vi "GraphView.vi"(1 "Increment":dbl, 2 "End":dbl, 3 "Start":dbl) -> (0 "Array":dbl[](array[numeric]))   [LabVIEW 2023]
panel:
  out "increment":dbl format="%#_4f"
  in  "stop":bool
  out "Waveform Graph":dbl[][](graph)
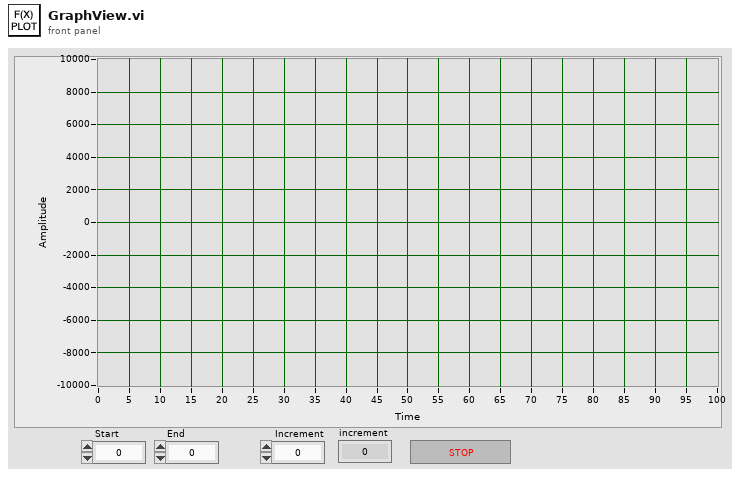
[diagram p1: front panel]
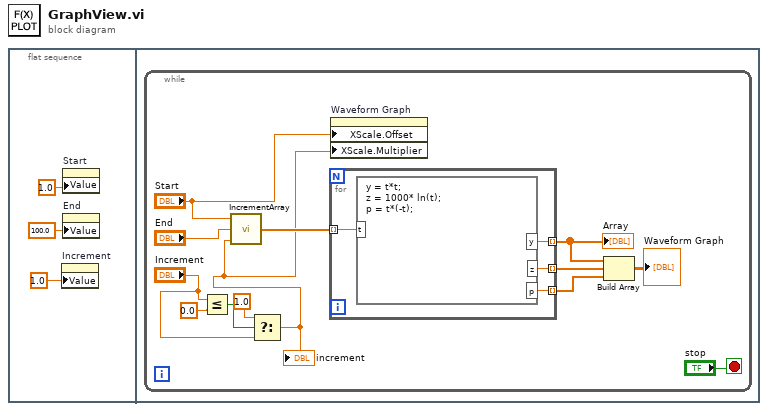
[diagram p0: block diagram]
diagram:
  n1 = flat-sequence {
    frame #0 {
      n2 = property on="Increment" class="DigNum (strict)"("Value"=1.0 ("End")) -> ()  [unwired: 2 in, 2 out]
      n3 = property on="Start" class="DigNum (strict)"("Value"=1.0 ("Start")) -> ()  [unwired: 2 in, 2 out]
      n4 = property on="End" class="DigNum (strict)"("Value"=100.0 ("End")) -> ()  [unwired: 2 in, 2 out]
    }
    frame #1 {
      n5 = while {
        stop <- "stop" stop-if-true
        n6 = Less Or Equal?(x="Increment", y=0.0) -> (x <= y?=w7:bool)
        n7 = Select(t=1.0, s=w7, f="Increment") -> (s? t:f=w4:dbl)
        "increment" <- w4
        n8 = call "IncrementArray.vi"("Increment"=w4, "End"="End", "Start"="Start") -> ("Array"=w15:dbl[])
        n9 = for {
          tunnel: w15 -> [w19] mode=indexing
          tunnel: [w20] -> w13 mode=indexing
          tunnel: [w18] -> w12 mode=indexing
          tunnel: [w17] -> w10 mode=indexing
          n10 = formula code="y = t*t;\nz = 1000* ln(t);\np = t*(-t);"("t"=w19) -> ("y"=w20:dbl, "z"=w18:dbl, "p"=w17:dbl)
        }
        "Array" <- w13
        n11 = property on="Waveform Graph" class="WFGraph (strict)"("XScale.Offset"="Start", "XScale.Multiplier"=w4) -> ()  [unwired: 2 in, 2 out]
        n12 = Build Array(w13, w12, w10) -> (→"Waveform Graph":dbl[][])
      }
    }
  }
